vi "Test 1 Serial Write Data is Written to Log.vi"(8 "error in (no error)":errorcluster, 11 "Test Case In":refnum<class "Serial Logging Decorator Test.lvclass">) -> (0 "error out":errorcluster, 3 "Test Case Out":refnum<class "Serial Logging Decorator Test.lvclass">)   [LabVIEW 2020, in "Serial Logging Decorator Test.lvclass"]
uses:
  Serial Logging Decorator Test.lvclass
  Serial Logging Decorator Test.lvclass/Serial Logging Decorator Test.ctl
  Serial Logging Decorator/Serial Logging Decorator.lvclass
  Log Mock/Mock Log.lvclass
  Serial/Serial.lvclass/Serial.lvclass
  Framework/Verifier/Verifier.lvclass
  C:/Program Files (x86)/National Instruments/LabVIEW 2020/vi.lib/Astemes/LUnit/Test Case.lvclass
  C:/Program Files (x86)/National Instruments/LabVIEW 2020/vi.lib/Astemes/LUnit/LUnit Runnable.lvclass
  C:/git/astemes-lmock/source/Examples/Serial Driver/Logging Decorator Test/Serial Logging Decorator Test.lvclass
  Framework/LMock API.lvlib
  C:/git/astemes-lmock/source/Framework/Mock/LMock Mock.lvclass
  C:/git/astemes-lmock/source/Examples/Serial Driver/Log Mock/Mock Log.lvclass
  C:/git/astemes-lmock/source/Examples/Serial Driver/Log/Log.lvclass
  Expectations/One/One Matching String Inputs.vi
  Expectations/One/One.lvlib
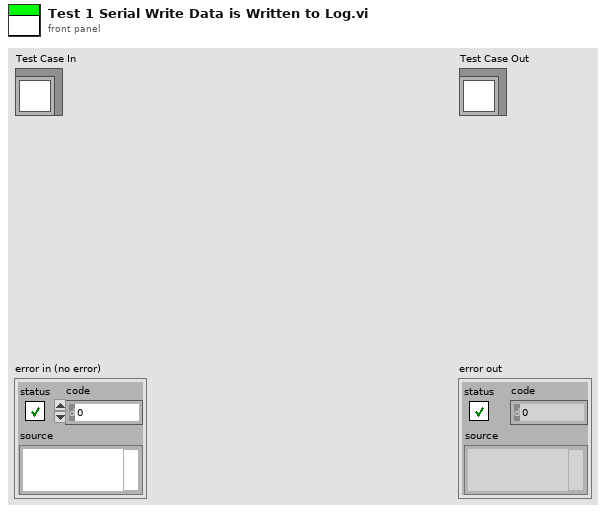
[diagram p1: front panel]
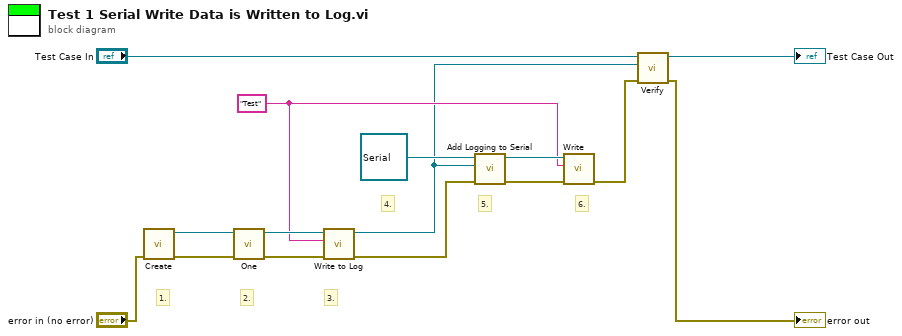
[diagram p0: block diagram]
diagram:
  w4 = "Test" ("Text to Write")
  # "6."
  # "5."
  # "4."
  # "3."
  # "2."
  # "1."
  n1 = call "Create.vi"("error in (no error)"="error in (no error)") -> ("error out"=w11:errorcluster, "Mock Class Generator out"=w12:refnum<class "Mock Log.lvclass">)  [unwired: 9 in]
  n2 = call-poly "One.vi"("error in (no error)"=w11, "Mock in"=w12) -> ("error out"=w9:errorcluster, "Mock out"=w10:refnum<class "Mock Log.lvclass">)  [unwired: 8 in]
  n3 = call-dynamic "Write to Log.vi"("error in (no error)"=w9, "Text to Write"=w4, "Log in"=w10) -> ("error out"=w5:errorcluster, "Log out"=w1:refnum<class "Mock Log.lvclass">)  [unwired: 7 in]
  n4 = call "Add Logging to Serial.vi"("error in (no error)"=w5, "Log Destination"=w1, "Serial"=refnum<class "Serial.lvclass"> refnum ("Serial.lvclass")) -> ("error out"=w6:errorcluster, "Serial with Logging"=w7:refnum<class "Serial.lvclass">)  [unwired: 7 in]
  n5 = call-dynamic "Write.vi"("error in (no error)"=w6, "write buffer"=w4, "Serial in"=w7) -> ("error out"=w2:errorcluster)  [unwired: 6 in, 2 out]
  n6 = call "Verify.vi"("error in (no error)"=w2, "Mock"=w1, "LUnit Test Case In"="Test Case In") -> ("error out"=→"error out":errorcluster, "LUnit Test Case Out"=→"Test Case Out":refnum<class "Serial Logging Decorator Test.lvclass">)  [unwired: 7 in]
